vi "main_draw_projector.vi"(5 "camera notifier in":refnum<notifier>, 6 "projector loop queue in":refnum<queue>, 7 "stimulus loop notifier in":refnum<notifier>, 8 "error in":errorcluster, 9 "stimulus saving buffer":T1[](array[typedef]), 10 "ProjectorScaledImage in":T1, 11 "ProjectorImage in":T1) -> (0 "error out":errorcluster)   [LabVIEW 2019]
uses:
  <vilib>/vision/Image Controls.llb/IMAQ Image.ctl
  FauxWorm.ctl
  ActiveTracksFunctionalGlobalOperations.ctl
  radiucenter2boundingbox.vi
  ParametersGlobal.vi
  DebugGlobal.vi
  rotate_and_reflect_point.vi
  StimulusObject.lvclass
  <vilib>/vision/NI_Vision_Development_Module.lvlib
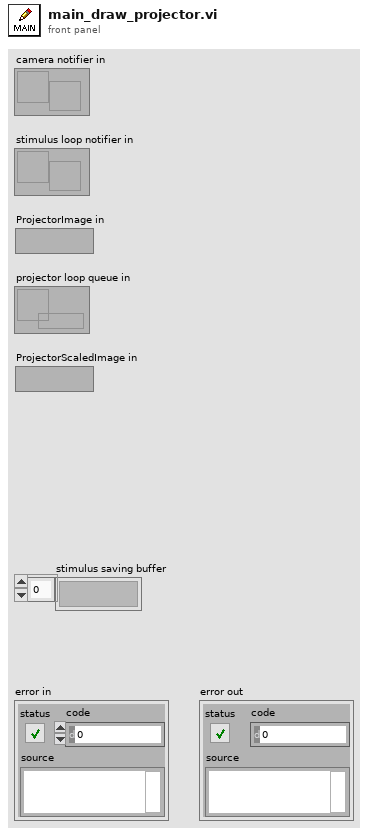
[diagram p1: front panel]
types:
  T1 = typedef "IMAQ Image.ctl" = refnum<image>
  T2 = typedef "Image Type" = u32
  T3 = typedef "FauxWorm.ctl" = cluster{"Centroid Position (Camera Pixel)":cluster{"X":sgl, "Y":sgl}, "Heading Direction (radians)":dbl, "Speed (mm/s)":sgl, "Length (mm)":sgl}
  T4 = typedef "ActiveTracksFunctionalGlobalOperations.ctl" = enum16{"Initialize", "ReadFullTrackGivenWormIndex", "WriteFullTrack", "ReadTrackSnippets", "WriteTrackGivenSnippets", "ReadStimulusSnippets", "StartNewTracksGivenSnippets", "EndTracksGivenSnippets", "WriteStimulusObjectGivenWormIndex", "CompleteAllActiveTracks", "ReturnAllActiveTrackIndecies"}
  T5 = typedef "StimulusSnippetCluster.ctl" = cluster{"Centerline Positions (Camera Pixel)":sgl[][], "Stimulus for frame (uW/mm^2)":sgl[]}
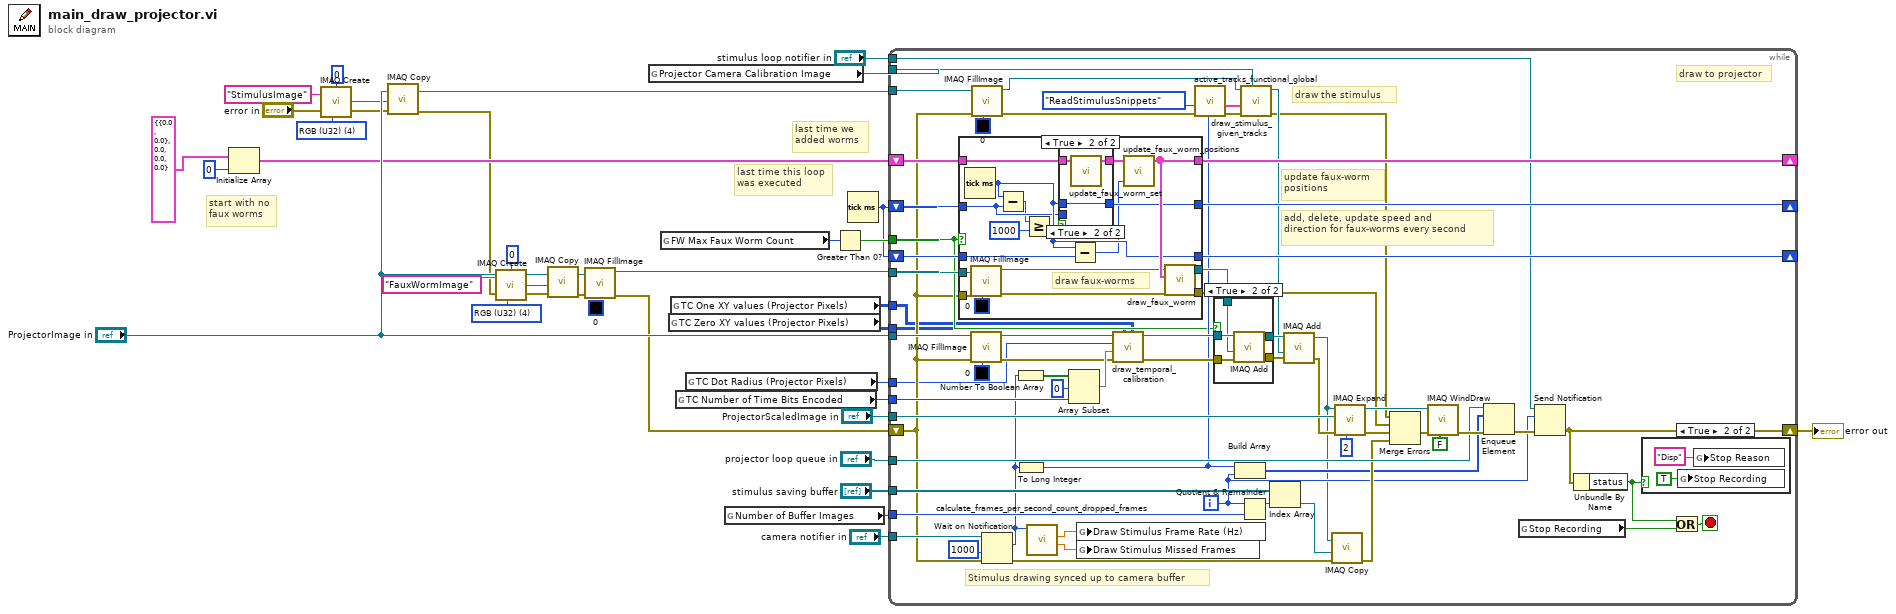
[diagram p0: block diagram]
diagram:
  (unwired) u32 0 ("Color Pixel Value")
  w27 = T2 4 items=["Grayscale (U8)", "Grayscale (I16)", "Grayscale (SGL)", "Complex (CSG)", "RGB (U32)", "HSL (U32)", "RGB (U64)", "Grayscale (U16)"] ("Image Type")
  w31 = T2 4 items=["Grayscale (U8)", "Grayscale (I16)", "Grayscale (SGL)", "Complex (CSG)", "RGB (U32)", "HSL (U32)", "RGB (U64)", "Grayscale (U16)"] ("Image Type")
  # "last time this loop\nwas executed"
  # "last time we\nadded worms"
  # "start with no\nfaux worms"
  n1 = Initialize Array(T3 {"Centroid Position (Camera Pixel)"={"X"=0.0, "Y"=0.0}, "Heading Direction (radians)"=0.0, "Speed (mm/s)"=0.0, "Length (mm)"=0.0} ("Faux Worm Properties"), 0) -> (w17:T3[])
  n2 = call "IMAQ Create"("Border Size"=0, "Image Name"="StimulusImage", "Image Type"=w27, "error in (no error)"="error in") -> ("New Image"=w21:T1, "error out"=w22:errorcluster)  [unwired: 1 in]
  n3 = call "IMAQ Copy"("error in (no error)"=w22, "Image Dst"=w21, "Image Src"="ProjectorImage in") -> ("error out"=w6:errorcluster, "Image Dst Out"=w35:T1)  [unwired: 3 in]
  n4 = call "IMAQ Create"("Border Size"=0, "Image Name"="FauxWormImage", "Image Type"=w31, "error in (no error)"=w6) -> ("New Image"=w23:T1, "error out"=w24:errorcluster)  [unwired: 1 in]
  n5 = call "IMAQ Copy"("error in (no error)"=w24, "Image Dst"=w23, "Image Src"="ProjectorImage in") -> ("error out"=w20:errorcluster, "Image Dst Out"=w19:T1)  [unwired: 3 in]
  n6 = call "IMAQ FillImage"("error in (no error)"=w20, "Image"=w19) -> ("error out"=w5:errorcluster, "Image Out"=w33:T1)  [unwired: 8 in]
  n7 = global read "ParametersGlobal.vi" "Projector Camera Calibration Image"() -> (w34:T1)
  n8 = global read "ParametersGlobal.vi" "FW Max Faux Worm Count"() -> (w18:i32)
  n9 = global read "ParametersGlobal.vi" "TC Zero XY values (Projector Pixels)"() -> (w2:i32[][])
  n10 = global read "ParametersGlobal.vi" "TC One XY values (Projector Pixels)"() -> (w1:i32[][])
  n11 = global read "ParametersGlobal.vi" "TC Number of Time Bits Encoded"() -> (w36:i32)
  n12 = global read "ParametersGlobal.vi" "TC Dot Radius (Projector Pixels)"() -> (w3:i32)
  n13 = global read "ParametersGlobal.vi" "Number of Buffer Images"() -> (w8:i32)
  n14 = Greater Than 0?(x=w18) -> (x > 0?=w32:bool)
  n15 = Tick Count (ms)() -> (millisecond timer value=w4:u32)
  n16 = while {
    tunnel: "ProjectorImage in" -> [w101]
    shift-right: [w53] -> w10
    shift-left: w5 -> [w40]
    shift-right: [w99] -> _
    shift-left: w17 -> [w100]
    tunnel: "camera notifier in" -> [w96]
    shift-right: [w93] -> _
    shift-left: w4 -> [w94]
    shift-right: [w95] -> _
    shift-left: w4 -> [w92]
    tunnel: w36 -> [w91]
    tunnel: w33 -> [w89]
    tunnel: "ProjectorScaledImage in" -> [w102]
    tunnel: w35 -> [w74]
    tunnel: w34 -> [w66]
    tunnel: "stimulus saving buffer" -> [w61]
    tunnel: w8 -> [w63]
    tunnel: "projector loop queue in" -> [w58]
    tunnel: "stimulus loop notifier in" -> [w52]
    tunnel: w32 -> [w47]
    tunnel: w3 -> [w39]
    tunnel: w2 -> [w38]
    tunnel: w1 -> [w37]
    i -> [w51]
    stop <- w90 stop-if-true
    # "draw to projector"
    # "draw the stimulus"
    # "Stimulus drawing synced up to camera buffer"
    # "add, delete, update speed and\ndirection for faux-worms every second"
    # "update faux-worm\npositions"
    n17 = case shown="True" w47 {
      tunnel: w100 -> [_ w131]
      tunnel: [_ w130] -> w99
      tunnel: [_ w129] -> w95
      tunnel: w94 -> [_ w128]
      tunnel: [_ w127] -> w93
      tunnel: w92 -> [_ w126]
      tunnel: w89 -> [w112 w125]
      tunnel: w40 -> [w113 w124]
      tunnel: [w112 w115] -> w79
      tunnel: [w113 w114] -> w77
      frame False {
      }
      frame True {
        # "draw faux-worms"
        n18 = Tick Count (ms)() -> (millisecond timer value=w129:u32)
        n19 = call "IMAQ FillImage"("Color Pixel Value"=u32 0, "error in (no error)"=w124, "Image"=w125) -> ("error out"=w117:errorcluster, "Image Out"=w116:T1)  [unwired: 7 in]
        n20 = Subtract(x=w129, y=w128) -> (x-y=w122:u32)
        n21 = Greater Or Equal?(x=w122, y=u32 1000) -> (x >= y?=w121:bool)
        n22 = case shown="True" w121 {
          tunnel: w131 -> [w133 w136]
          tunnel: [w133 w135] -> w123
          tunnel: w129 -> [_ w134]
          tunnel: [w132 w134] -> w127
          tunnel: w128 -> [w132 _]
          frame False {
          }
          frame True {
            n23 = call "update_faux_worm_set.vi"("Worms to Draw"=w136) -> ("Worms to Draw Updated"=w135:T3[])  [unwired: 4 in]
          }
        }
        n24 = Subtract(x=w129, y=w126) -> (x-y=w119:u32)
        n25 = call "update_faux_worm_positions.vi"("Update Time (ms)"=w119, "Worms to Draw"=w123) -> ("Worms to Draw Updated"=w130:T3[])  [unwired: 3 in]
        n26 = call "draw_faux_worm.vi"("error in (no error)"=w117, "Worms to Draw"=w130, "Image in"=w116) -> ("error out"=w114:errorcluster, "Image out"=w115:T1)  [unwired: 6 in]
      }
    }
    n27 = call "IMAQ FillImage"("Color Pixel Value"=u32 0, "error in (no error)"=w40, "Image"=w101) -> ("error out"=w83:errorcluster, "Image Out"=w82:T1)  [unwired: 7 in]
    n28 = call "IMAQ FillImage"("Color Pixel Value"=u32 0, "error in (no error)"=w40, "Image"=w74) -> ("error out"=w69:errorcluster, "Image Out"=w73:T1)  [unwired: 7 in]
    n29 = Wait on Notification(notifier=w96, timeout in ms (-1)=1000, error in (no error)=w40) -> (notification=w49:u32, error out=w56:errorcluster)  [unwired: 1 in, 2 out]
    n30 = Number To Boolean Array(number=w49) -> (Boolean array=w85:bool[])
    n31 = To Long Integer(number=w49) -> (32bit integer=w50:i32)
    n32 = call "calculate_frames_per_second_count_dropped_frames.vi"("Buffer Number"=w49) -> ("Missed Frames"=w42:dbl, "Processed Frames/s"=w43:dbl)  [unwired: 8 in, 1 out]
    n33 = Array Subset(array=w85, index=0, length=w91) -> (w86:bool[])
    n34 = global write "DebugGlobal.vi" "Draw Stimulus Frame Rate (Hz)"(w43) -> ()
    n35 = global write "DebugGlobal.vi" "Draw Stimulus Missed Frames"(w42) -> ()
    n36 = call "draw_temporal_calibration.vi"("TC One XY values (Projector Pixels)"=w37, "TC Zero XY values (Projector Pixels)"=w38, "error in (no error)"=w83, "Buffer  Bits To Be Encoded"=w86, "TC Dot Radius (Projector Pixels)"=w39, "Image in"=w82) -> ("error out"=w81:errorcluster, "Image Out"=w80:T1)  [unwired: 3 in]
    n37 = call "active_tracks_functional_global.vi"("Camera Frame In"=w50, "error in"=w69, "Operations"=ActiveTracksFunctionalGlobalOperations."ReadStimulusSnippets") -> ("error out"=w68:errorcluster, "Stimulus Snippets Out"=w65:T5[])  [unwired: 4 in, 3 out]
    n38 = case shown="True" w47 {
      tunnel: w81 -> [w105 w111]
      tunnel: w80 -> [w106 w110]
      tunnel: w79 -> [_ w109]
      tunnel: [w105 w108] -> w72
      tunnel: [w106 w107] -> w71
      frame False {
      }
      frame True {
        n39 = call "IMAQ Add"("Image Src A"=w110, "Image Src B"=w109, "error in (no error)"=w111) -> ("Image Dst Out"=w107:T1, "error out"=w108:errorcluster)  [unwired: 4 in]
      }
    }
    n40 = Build Array(w50, w51) -> (w48:i32[])
    n41 = Quotient & Remainder(x=w51, y=w63) -> (x-y*floor(x/y)=w62:i32)  [unwired: 1 out]
    n42 = call "draw_stimulus_given_tracks.vi"("Stimulus Image In"=w73, "Stimulus Snippet Array"=w65, "error in (no error)"=w68, "CalibrationImage"=w66) -> ("Stimulus Image Out"=w70:T1, "error out"=w64:errorcluster)  [unwired: 5 in]
    n43 = Index Array(array=w61, index=w62) -> (element=w60:T1)
    n44 = call "IMAQ Add"("Image Src A"=w71, "Image Src B"=w70, "error in (no error)"=w72) -> ("Image Dst Out"=w46:T1, "error out"=w57:errorcluster)  [unwired: 4 in]
    n45 = call "IMAQ Copy"("error in (no error)"=w56, "Image Dst"=w60, "Image Src"=w46) -> ("error out"=w55:errorcluster)  [unwired: 3 in, 1 out]
    n46 = call "IMAQ Expand"("Y Duplication Step"=2, "error in (no error)"=w57, "Image Dst"=w102, "Image Src"=w46) -> ("error out"=w78:errorcluster, "Image Dst Out"=w97:T1)  [unwired: 6 in]
    n47 = Merge Errors(w64, w77, w78, w55) -> (w98:errorcluster)
    n48 = call "IMAQ WindDraw"("Resize to Image Size? (Y)"=FALSE, "error in (no error)"=w98, "Image"=w97) -> ("error out"=w59:errorcluster)  [unwired: 7 in, 1 out]
    n49 = Enqueue Element(queue=w58, element=w48, error in (no error)=w59) -> (error out=w54:errorcluster)  [unwired: 1 in, 2 out]
    n50 = global read "DebugGlobal.vi" "Stop Recording"() -> (w44:bool)
    n51 = Send Notification(notification=w51, notifier=w52, error in (no error)=w54) -> (error out=w53:errorcluster)  [unwired: 1 out]
    n52 = Unbundle By Name(w53) -> ("status"=w45:bool)
    n53 = case shown="True" w45 {
      frame False {
      }
      frame True {
        n54 = global write "DebugGlobal.vi" "Stop Recording"(TRUE ("stop")) -> ()
        n55 = global write "DebugGlobal.vi" "Stop Reason"("Disp" ("Stop Debug")) -> ()
      }
    }
    n56 = Or(x=w45, y=w44) -> (x .or. y?=w90:bool)
  }
  "error out" <- w10
